vi "testing_cam_ai_ao.vi"() -> ()   [LabVIEW 2015]
uses:
  <vilib>/Platform/storage/lvStorage.llb/_openFunction.ctl
  <vilib>/addons/h5labview2/file/H5Fmode.ctl
  <vilib>/DAQmx/write.llb/DAQmx Write (Analog Wfm 1Chan NSamp).vi
  <vilib>/DAQmx/write.llb/DAQmx Write (Digital Bool 1Line 1Point).vi
  <vilib>/DAQmx/read.llb/DAQmx Read (Analog 1D Wfm NChan NSamp).vi
  <vilib>/DAQmx/create/channels.llb/DAQmx Create Channel (AI-Voltage-Basic).vi
  <vilib>/DAQmx/configure/timing.llb/DAQmx Timing (Sample Clock).vi
  <vilib>/DAQmx/create/channels.llb/DAQmx Create Channel (DO-Digital Output).vi
  <vilib>/DAQmx/create/channels.llb/DAQmx Create Channel (AO-Voltage-Basic).vi
  <vilib>/Platform/storage/lvStorage.llb/_openStorageWithRootAutoDetect.vi
  <vilib>/Platform/storage/lvStorage.llb/xStorage/xStorageSupp/ErrorOut.vi
  <vilib>/Platform/storage/lvStorage.llb/_queryPropPoly.vi
  <vilib>/Platform/storage/lvStorage.llb/_queryPropString.vi
  <vilib>/Platform/storage/lvStorage.llb/_queryGenericObjects.vi
  <vilib>/Platform/storage/lvStorage.llb/_loadAllDdt.vi
  <vilib>/DAQmx/miscellaneous.llb/DAQmx Fill In Error Info.vi
  <vilib>/addons/h5labview2/base/lib_path.vi
  <vilib>/addons/h5labview2/base/H5Equery.vi
  <vilib>/addons/h5labview2/base/hid_t.ctl
  <vilib>/Platform/storage/lvStorage.llb/xStorage/Open Data Storage/Open Data Storage.xnode
  <vilib>/Platform/storage/lvStorage.llb/xStorage/Read Data/Read Data.xnode
  <vilib>/addons/h5labview2/attrib/H5Awrite.llb/H5Awrite.xnode
  <vilib>/addons/h5labview2/dataset/H5Dwrite.llb/H5Dwrite.xnode
  <resource>/objmgr/daqmx.rc
  <vilib>/addons/h5labview2/file/H5F.lvlib
  <vilib>/addons/h5labview2/group/H5G.lvlib
  <vilib>/addons/h5labview2/dataset/H5D.lvlib
  <vilib>/addons/h5labview2/space/H5S.lvlib
panel:
  out "replaced?":bool
  out "error out 4":errorcluster
  out "error out 3":errorcluster
  out "Timeseries Base Filename 2":string
  out "Acquiring Frames":bool
  out "DataPlugin name out":string
  in  "Path":path=path "E:/code/labview-phys-io/001_pure_sines_151013_10Hz.mat"
  out "Actual Sample Rate 2":dbl=1000.0 format="%0.2f"
  out "Stop DAC":bool
  out "n loop":dbl
  out "Measurement":waveform(dbl)[](graph)
  out "error out 2":errorcluster
  out "error out":errorcluster
  in  "Frames":i32=100
  out "Timeseries save path":path
  out "Timeseries Base Filename":string
  out "Image":u16[][](graph)
  in  "stop":bool
  out "Frames Recorded":i32
  in  "Start Button":bool
  out "No Cam Probs":bool
  out "DCAM Ver.":string
  out "Library Ver.":string
  out "Model":string
  out "Camera ID":string
  out "Firmware":string
  out "Actual Sample Rate":dbl=1000.0 format="%0.2f"
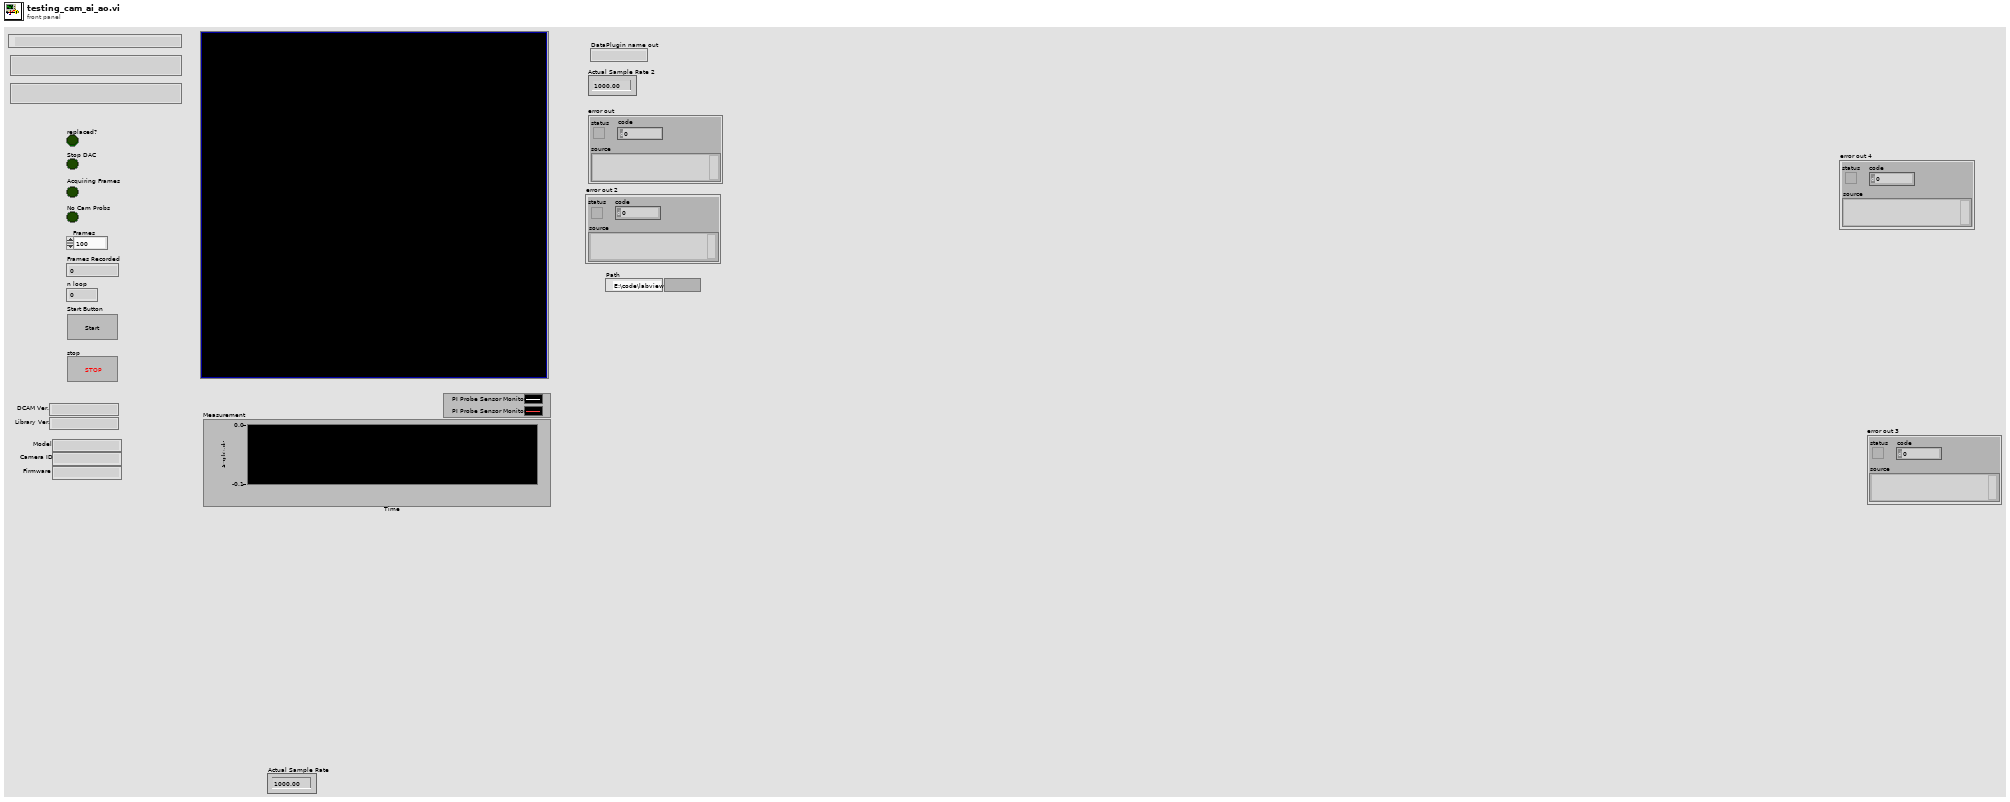
[diagram p1: front panel]
types:
  T1 = cluster{"Capture Library":string, "DCAM-API":string}
  T2 = cluster{"Model":string, "Camera ID":string, "Firmware":string}
  T3 = cluster{"height":u32, "width":u32, "datatype":u32}
  T4 = typedef "H5F.lvlib/H5Fmode.ctl" = enum16{"read-only", "read-write", "overwrite", "create new", "open or create"}
  T5 = typedef "hid_t.ctl" = i32
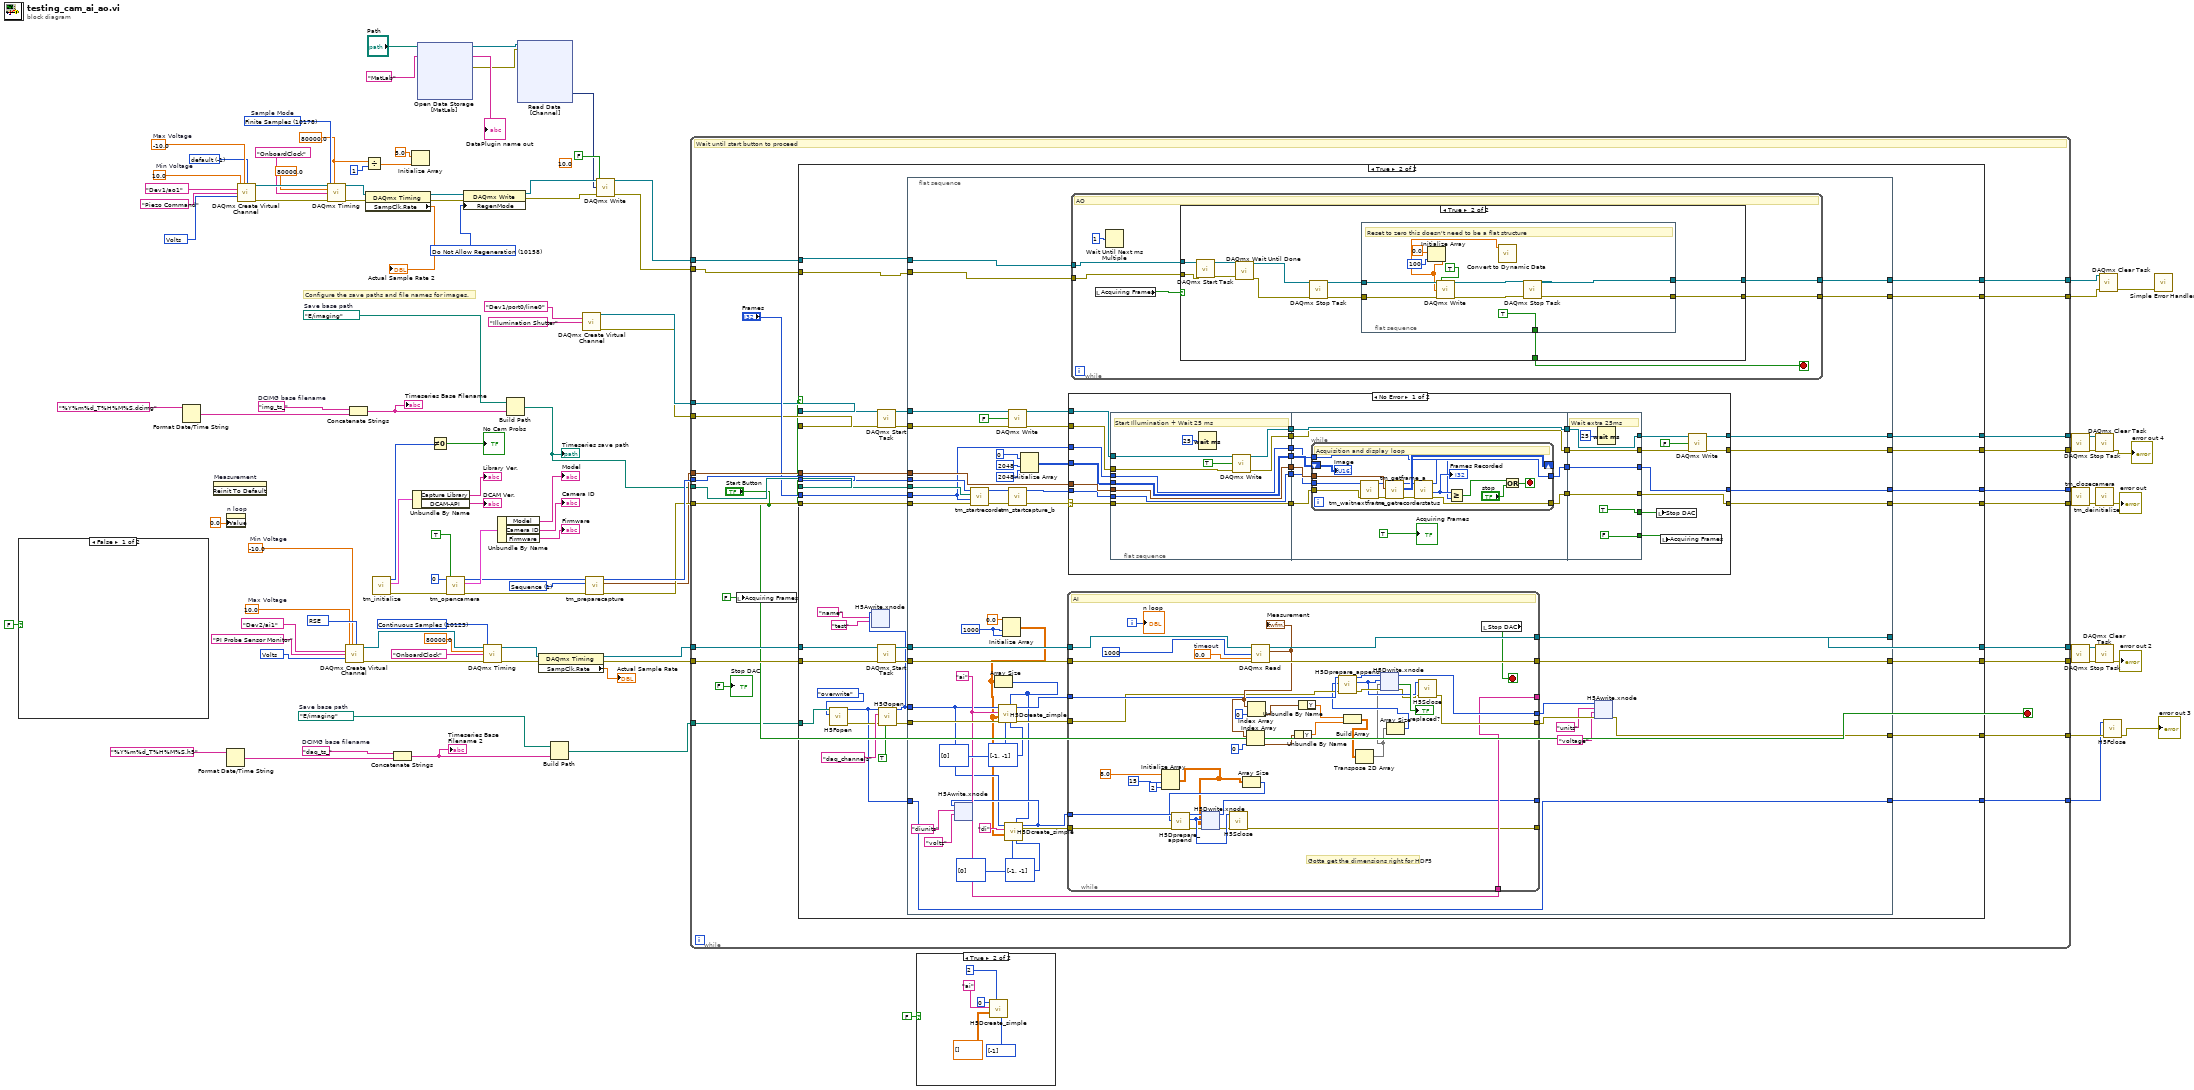
[diagram p0: block diagram]
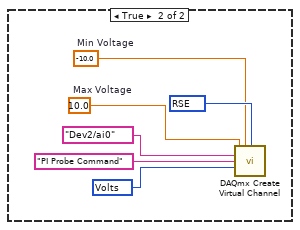
[diagram p3: hidden frame]
diagram:
  w9 = "daq_ts_"  # DCIMG base filename
  w12 = path "E:/imaging"  # Save base path
  w24 = 10158 items=["Allow Regeneration"=10097, "Do Not Allow Regeneration"=10158] ("RegenMode")
  w31 = 80000.0
  (unwired) 10.0
  w38 = 10178 items=["Finite Samples"=10178, "Continuous Samples"=10123, "Hardware Timed Single Point"=12522]  # Sample Mode
  w39 = -1 items=["default"=-1, "RSE"=10083, "NRSE"=10078, "Differential"=10106, "Pseudodifferential"=12529] ("input terminal configuration")
  w40 = 10348 items=["Volts"=10348, "From Custom Scale"=10065] ("units")
  w44 = 10.0  # Min Voltage
  w43 = -10.0  # Max Voltage
  w59 = 1 items=["Snap", "Sequence"] ("Capture mode")
  w67 = 10123 items=["Finite Samples"=10178, "Continuous Samples"=10123] ("sample mode")
  w77 = 10348 items=["Volts"=10348, "From Custom Scale"=10065] ("units")
  w76 = 10083 items=["default"=-1, "RSE"=10083, "NRSE"=10078, "Differential"=10106, "Pseudodifferential"=12529] ("input terminal configuration")
  w74 = -10.0  # Min Voltage
  w75 = 10.0  # Max Voltage
  w91 = "img_ts_"  # DCIMG base filename
  w94 = path "E:/imaging"  # Save base path
  # "Configure the save paths and file names for images."
  n1 = case shown="False" FALSE {
    frame False {
    }
    frame True {
      w109 = 10348 items=["Volts"=10348, "From Custom Scale"=10065] ("units")
      w108 = 10083 items=["default"=-1, "RSE"=10083, "NRSE"=10078, "Differential"=10106, "Pseudodifferential"=12529] ("input terminal configuration")
      w106 = -10.0  # Min Voltage
      w107 = 10.0  # Max Voltage
      n2 = call-poly <vilib>:"DAQmx Create Virtual Channel.vi"("maximum value"=w107, "minimum value"=w106, "input terminal configuration"=w108, "physical channels"=tag "Dev2/ai0" ("DAQmx Physical Channel"), "name to assign"="PI Probe Command", "units"=w109) -> ()  [unwired: 8 in, 2 out]
    }
  }
  n3 = Format Date/Time String(time format string (%c)="%Y%m%d_T%H%M%S.dcimg" ("name or relative path")) -> (date/time string=w92:string)  [unwired: 2 in]
  n4 = invoke on="Measurement" class="WFChart (strict)" method="Reinit To Default"() -> ()  [unwired: 3 in, 3 out]
  n5 = property on="n loop" class="DigNum (strict)"("Value"=0.0 ("n loop")) -> ()  [unwired: 2 in, 2 out]
  n6 = Format Date/Time String(time format string (%c)="%Y%m%d_T%H%M%S.h5" ("name or relative path")) -> (date/time string=w10:string)  [unwired: 2 in]
  n7 = call-poly <vilib>:"DAQmx Create Virtual Channel.vi"("maximum value"=w44, "minimum value"=w43, "output terminal configuration"=w39, "physical channels"=tag "Dev1/ao1" ("DAQmx Physical Channel"), "name to assign"="Piezo Command", "units"=w40) -> ("task out"=w46:refnum<k21>, "error out"=w47:errorcluster)  [unwired: 8 in]
  n8 = call-poly <vilib>:"DAQmx Timing.vi"("task/channels in"=w46, "sample mode"=w38, "samples per channel"=w31, "rate"=80000.0, "source"=tag "OnboardClock" ("Sample Clock Source"), "error in"=w47) -> ("task out"=w36:refnum<k21>, "error out"=w35:errorcluster)  [unwired: 8 in]
  n9 = call-poly <vilib>:"DAQmx Create Virtual Channel.vi"("maximum value"=w75, "minimum value"=w74, "input terminal configuration"=w76, "physical channels"=tag "Dev2/ai1" ("DAQmx Physical Channel"), "name to assign"="PI Probe Sensor Monitor", "units"=w77) -> ("task out"=w69:refnum<k21>, "error out"=w68:errorcluster)  [unwired: 8 in]
  n10 = Concatenate Strings(w91, w92) -> (w90:string)
  "Timeseries Base Filename" <- w90
  n11 = Divide(x=w31, y=1) -> (x/y=w30:dbl)
  n12 = property class="DAQmx Timing"(reference=w36, error in=w35) -> (reference out=w28:refnum<k21>, error out=w27:errorcluster, "SampClk.Rate"=→"Actual Sample Rate 2":dbl)
  n13 = call <userlib>:"tm_initialize.vi"() -> ("error out"=w100:errorcluster, "Version Info"=w104:T1, "Number Of Cameras"=w105:u32)  [unwired: 8 in, 1 out]
  n14 = Concatenate Strings(w9, w10) -> (w8:string)
  "Timeseries Base Filename 2" <- w8
  n15 = Initialize Array(5.0 ("element"), w30) -> ()  [unwired: 1 out]
  n16 = Unbundle By Name(w104) -> ("Capture Library"=→"Library Ver.":string, "DCAM-API"=→"DCAM Ver.":string)
  n17 = xnode "Open Data Storage\n[MatLab]"("file path"="Path", "DataPlugin name"="MatLab") -> ("storage refnum (file)"=w22:refnum<k20>, "DataPlugin name out"=→"DataPlugin name out":string, "error out"=w19:errorcluster)  [unwired: 3 in]
  n18 = Not Equal To 0?(x=w105) -> (x != 0?=→"No Cam Probs":bool)
  n19 = call <userlib>:"tm_opencamera.vi"("Force Open"=TRUE, "error in (no error)"=w100, "Camera Index"=0) -> ("error out"=w57:errorcluster, "Camera Details"=w60:T2, "Handle out"=w58:u32)  [unwired: 6 in]
  n20 = property class="DAQmx Write"(reference=w28, error in=w27, "RegenMode"=w24) -> (reference out=w26:refnum<k21>, error out=w25:errorcluster)
  n21 = call-poly <vilib>:"DAQmx Timing.vi"("task/channels in"=w69, "sample mode"=w67, "rate"=80000.0, "source"=tag "OnboardClock" ("Sample Clock Source"), "error in"=w68) -> ("task out"=w73:refnum<k21>, "error out"=w72:errorcluster)  [unwired: 9 in]
  n22 = Unbundle By Name(w60) -> ("Model"=→"Model":string, "Camera ID"=→"Camera ID":string, "Firmware"=→"Firmware":string)
  n23 = Build Path(base path=w94, name or relative path=w90) -> (appended path=w89:path)
  "Timeseries save path" <- w89
  n24 = xnode "Read Data\n[Channel]"("storage refnum (file)"=w22, "error in"=w19) -> ("Signal"=w20:dynamicdata)  [unwired: 2 in, 3 out]
  n25 = property class="DAQmx Timing"(reference=w73, error in=w72) -> (reference out=w96:refnum<k21>, error out=w95:errorcluster, "SampClk.Rate"=→"Actual Sample Rate":dbl)
  n26 = Build Path(base path=w12, name or relative path=w8) -> (appended path=w7:path)
  n27 = call-poly <vilib>:"DAQmx Create Virtual Channel.vi"("lines"=tag "Dev1/port0/line0" ("DAQmx Physical Channel"), "name to assign"="Illumination Shutter") -> ("task out"=w53:refnum<k21>, "error out"=w52:errorcluster)  [unwired: 12 in]
  n28 = call <userlib>:"tm_preparecapture.vi"("error in (no error)"=w57, "Capture mode"=w59, "Handle in"=w58) -> ("error out"=w98:errorcluster, "Buffer Info"=w97:T3, "Handle out"=w99:u32)  [unwired: 5 in, 1 out]
  n29 = call-poly <vilib>:"DAQmx Write.vi"("task/channels in"=w26, "auto start"=FALSE, "data"=w20, "error in"=w25) -> ("task out"=w17:refnum<k21>, "error out"=w16:errorcluster)  [unwired: 9 in, 1 out]
  n30 = while {
    tunnel: w99 -> [w135]
    tunnel: w98 -> [w133]
    tunnel: w97 -> [w134]
    tunnel: w96 -> [w129]
    tunnel: w95 -> [w128]
    tunnel: w89 -> [w136]
    tunnel: [w131] -> w86
    tunnel: [w130] -> w85
    tunnel: [w127] -> w81
    tunnel: [w126] -> w80
    tunnel: w53 -> [w124]
    tunnel: w52 -> [w123]
    tunnel: [w122] -> w49
    tunnel: [w121] -> w48
    tunnel: w17 -> [w118]
    tunnel: w16 -> [w119]
    tunnel: [w116] -> w14
    tunnel: [w115] -> w13
    tunnel: w7 -> [w114]
    tunnel: [w113] -> w6
    tunnel: [w112] -> w1
    stop <- "Start Button" stop-if-true
    # "Wait until start button to proceed"
    n31 = local write "Acquiring Frames"(FALSE ("Acquiring Frames")) -> ()
    n32 = case shown="True" "Start Button" {
      tunnel: w136 -> [_ w179]
      tunnel: w135 -> [w142 w178]
      tunnel: w134 -> [_ w177]
      tunnel: w133 -> [w141 w176]
      tunnel: "Frames" -> [_ w175]
      tunnel: [w142 w174] -> w131
      tunnel: [w141 w173] -> w130
      tunnel: w129 -> [w144 w172]
      tunnel: w128 -> [w143 w171]
      tunnel: [w144 w168] -> w127
      tunnel: [w143 w167] -> w126
      tunnel: w124 -> [w140 w166]
      tunnel: w123 -> [w139 w165]
      tunnel: [w140 w162] -> w122
      tunnel: [w139 w161] -> w121
      tunnel: w119 -> [w138 w159]
      tunnel: w118 -> [w137 w160]
      tunnel: [w137 w158] -> w116
      tunnel: [w138 w157] -> w115
      tunnel: w114 -> [_ w156]
      tunnel: [_ w154] -> w113
      tunnel: [_ w149] -> w112
      frame False {
      }
      frame True {
        n33 = call <vilib>:"H5Fopen.vi"("mode (read-only)"=H5Fmode."overwrite" ("mode"), "path"=w156) -> ("error out"=w151:errorcluster, "ref out"=w148:T5)  [unwired: 8 in]
        n34 = call <vilib>:"DAQmx Start Task.vi"("task/channels in"=w166, "error in"=w165) -> ("task out"=w163:refnum<k21>, "error out"=w164:errorcluster)  [unwired: 12 in]
        n35 = call <vilib>:"DAQmx Start Task.vi"("task/channels in"=w172, "error in"=w171) -> ("task out"=w170:refnum<k21>, "error out"=w169:errorcluster)  [unwired: 12 in]
        n36 = call <vilib>:"H5Gopen.vi"("create? (F)"=TRUE, "error in (no error)"=w151, "name"="daq_channels", "ref in"=w148) -> ("error out"=w150:errorcluster, "group out"=w147:T5)  [unwired: 6 in]
        n37 = xnode "H5Awrite.xnode"("data"="test" ("name"), "attrib name"="name" ("name"), "ref in"=w147) -> ()  [unwired: 4 in, 3 out]
        n38 = flat-sequence {
          tunnel: w179 -> [w251]
          tunnel: w178 -> [w250]
          tunnel: w177 -> [w249]
          tunnel: w176 -> [w248]
          tunnel: w175 -> [w247]
          tunnel: w170 -> [w236]
          tunnel: w169 -> [w235]
          tunnel: w163 -> [w231]
          tunnel: w164 -> [w230]
          tunnel: [w246] -> w174
          tunnel: [w245] -> w173
          tunnel: [w234] -> w168
          tunnel: [w233] -> w167
          tunnel: [w227] -> w162
          tunnel: [w226] -> w161
          tunnel: w159 -> [w225]
          tunnel: w160 -> [w224]
          tunnel: [w223] -> w158
          tunnel: [w222] -> w157
          tunnel: w150 -> [w213]
          tunnel: [w219] -> w154
          tunnel: w148 -> [w216]
          tunnel: [w216] -> w149
          tunnel: w147 -> [w201]
          frame #0 {
            w200 = 1000 ("dimension size")
            w211 = "ai"
            n39 = call <userlib>:"tm_startrecorder.vi"("error in (no error)"=w248, "frames"=w247, "File"=w251, "Handle in"=w250) -> ("error out"=w239:errorcluster, "Handle out"=w238:u32)  [unwired: 6 in]
            n40 = Initialize Array(0.0 ("element"), w200, w200) -> (w199:dbl[][])
            n41 = Array Size(array=w199) -> (size(s)=w198:i32[])
            n42 = call <vilib>:"H5Dcreate_simple.vi"("max size"=i32[] [-1, -1], "chunk size"=w198, "initial size"=i32[] [0], "error in (no error)"=w213, "type in"=w199, "name"=w211, "ref in"=w201) -> ("error out"=w202:errorcluster, "dset out"=w212:T5)  [unwired: 3 in]
            n43 = call <vilib>:"H5Dcreate_simple.vi"("max size"=i32[] [-1, -1], "chunk size"=w198, "initial size"=i32[] [0], "type in"=w199, "name"="di", "ref in"=w201) -> ("error out"=w206:errorcluster, "dset out"=w203:T5)  [unwired: 4 in]
            n44 = xnode "H5Awrite.xnode"("data"="voltz" ("name"), "attrib name"="diunits" ("name"), "ref in"=w203) -> ()  [unwired: 4 in, 3 out]
            n45 = call-poly <vilib>:"DAQmx Write.vi"("task/channels in"=w231, "data"=FALSE, "error in"=w230) -> ("task out"=w229:refnum<k21>, "error out"=w228:errorcluster)  [unwired: 10 in, 1 out]
            n46 = call <userlib>:"tm_startcapture_b.vi"("error in (no error)"=w239, "Handle in"=w238) -> ("error out"=w237:errorcluster, "Handle out"=w244:u32)  [unwired: 8 in]
            n47 = Initialize Array(u16 0 ("element"), 2048 ("dimension size"), 2048 ("dimension size")) -> (w240:u16[][])
            n48 = while {
              tunnel: w235 -> [w359]
              tunnel: w236 -> [w358]
              tunnel: [w357] -> w234
              tunnel: [w356] -> w233
              tunnel: [w337] -> _
              tunnel: [w342] -> w220
              tunnel: [w340] -> w221
              tunnel: w212 -> [w339]
              tunnel: w202 -> [w338]
              tunnel: w211 -> [w337]
              tunnel: w206 -> [w332]
              tunnel: w203 -> [w331]
              tunnel: [w329] -> _
              tunnel: [w328] -> _
              i -> [w352]
              stop <- w353 stop-if-true
              w355 = 0.0  # timeout
              # "Gotta get the dimensions right for HDF5"
              # "AI"
              n49 = Initialize Array(8.0 ("element"), 15 ("dimension size"), 2 ("dimension size")) -> (w319:dbl[][])
              n50 = Array Size(array=w319) -> (size(s)=w322:i32[])
              n51 = call <vilib>:"H5Dprepare_append.vi"("error in (no error)"=w332, "append dims"=w322, "dset in"=w331) -> ("error out"=w333:errorcluster, "space out"=w335:T5, "dset out"=w336:T5)  [unwired: 6 in]
              n52 = xnode "H5Dwrite.xnode"("error in (no error)"=w333, "data"=w319, "file space"=w335, "ref in"=w336) -> ("error out"=w334:errorcluster, "ref out"=w329:T5)  [unwired: 3 in, 1 out]
              n53 = call <vilib>:"H5Sclose.vi"("error in (no error)"=w334, "space in"=w335) -> ("error out"=w328:errorcluster)  [unwired: 9 in]
              n54 = call-poly <vilib>:"DAQmx Read.vi"("task/channels in"=w358, "number of samples per channel"=1000 ("Samples to Read"), "timeout"=w355, "error in"=w359) -> ("task out"=w357:refnum<k21>, "data"=w348:waveform(dbl)[], "error out"=w356:errorcluster)  [unwired: 9 in]
              "Measurement" <- w348
              n55 = Index Array(array=w348, index=0) -> (element=w347:waveform(dbl))
              n56 = Index Array(array=w348, index=0) -> (element=w350:waveform(dbl))
              n57 = Unbundle By Name(w347) -> ("Y"=w326:dbl[])
              n58 = Unbundle By Name(w350) -> ("Y"=w327:dbl[])
              n59 = Build Array(w327, w326) -> (w324:dbl[][])
              n60 = Transpose 2D Array(2D array=w324) -> (transposed array=w323:dbl[][])
              n61 = Array Size(array=w323) -> (size(s)=w325:i32[])
              n62 = call <vilib>:"H5Dprepare_append.vi"("error in (no error)"=w338, "append dims"=w325, "dset in"=w339) -> ("error out"=w344:errorcluster, "space out"=w343:T5, "dset out"=w345:T5)  [unwired: 6 in]
              n63 = xnode "H5Dwrite.xnode"("error in (no error)"=w344, "data"=w323, "file space"=w343, "ref in"=w345) -> ("error out"=w341:errorcluster, "replaced?"=→"replaced?":bool, "ref out"=w342:T5)  [unwired: 3 in]
              n64 = call <vilib>:"H5Sclose.vi"("error in (no error)"=w341, "space in"=w343) -> ("error out"=w340:errorcluster)  [unwired: 9 in]
              n65 = local read "Stop DAC"() -> (w353:bool)
              "n loop" <- w352
            }
            n66 = case shown="No Error" w237 {
              selector: w237 -> [w416 w470]
              tunnel: w249 -> [w422 _]
              tunnel: w244 -> [w421 w469]
              tunnel: w240 -> [w420 _]
              tunnel: [w419 w469] -> w246
              tunnel: [w418 w470] -> w245
              tunnel: w247 -> [w417 _]
              tunnel: w229 -> [w407 w467]
              tunnel: w228 -> [w406 w468]
              tunnel: [w398 w467] -> w227
              tunnel: [w397 w468] -> w226
              frame No Error {
                n67 = flat-sequence {
                  tunnel: w416 -> [w429]
                  tunnel: w417 -> [w430]
                  tunnel: w420 -> [w431]
                  tunnel: w421 -> [w432]
                  tunnel: w422 -> [w433]
                  tunnel: [w433] -> w412
                  tunnel: [w432] -> w411
                  tunnel: [w431] -> w410
                  tunnel: [w430] -> w409
                  tunnel: [w429] -> w408
                  tunnel: w407 -> [w426]
                  tunnel: w406 -> [w425]
                  tunnel: [w424] -> w404
                  tunnel: [w423] -> w399
                  tunnel: [w440] -> w414
                  tunnel: [w439] -> w413
                  tunnel: w412 -> [w443]
                  tunnel: w411 -> [w442]
                  tunnel: w410 -> [w441]
                  tunnel: w409 -> [w438]
                  tunnel: w408 -> [w437]
                  tunnel: w404 -> [w436]
                  tunnel: [w436] -> w403
                  tunnel: [w435] -> w400
                  tunnel: w399 -> [w435]
                  tunnel: [TRUE] -> w415
                  tunnel: [w465] -> w418
                  tunnel: [w466] -> w419
                  tunnel: w414 -> [w466]
                  tunnel: w413 -> [w465]
                  tunnel: w403 -> [w462]
                  tunnel: [w462] -> w402
                  tunnel: [w461] -> w401
                  tunnel: w400 -> [w461]
                  tunnel: [FALSE] -> w396
                  frame #0 {
                    # "Start Illumination + Wait 25 ms"
                    n68 = Wait (ms)(milliseconds to wait=u32 25) -> ()  [unwired: 1 out]
                    n69 = call-poly <vilib>:"DAQmx Write.vi"("task/channels in"=w426, "data"=TRUE, "error in"=w425) -> ("task out"=w424:refnum<k21>, "error out"=w423:errorcluster)  [unwired: 10 in, 1 out]
                  }
                  frame #1 {
                    n70 = while {
                      tunnel: w443 -> [w459]
                      tunnel: w442 -> [w458]
                      tunnel: w437 -> [w455]
                      shift-right: [w453] -> _
                      shift-left: w441 -> [w454]
                      tunnel: [w450] -> w440
                      tunnel: [w449] -> w439
                      tunnel: w438 -> [w444]
                      stop <- w447 stop-if-true
                      # "Acquisition and display loop"
                      n71 = call <userlib>:"tm_waitnextframe.vi"("error in (no error)"=w455, "Handle in"=w458) -> ("error out"=w456:errorcluster, "Handle out"=w457:u32)  [unwired: 6 in, 2 out]
                      n72 = call <userlib>:"tm_getframe_a.vi"("error in (no error)"=w456, "Buffer Info"=w459, "Handle in"=w457) -> ("error out"=w452:errorcluster, "Data 16"=w453:u16[][], "Handle out"=w451:u32)  [unwired: 4 in, 2 out]
                      n73 = call <userlib>:"tm_getrecorderstatus.vi"("error in (no error)"=w452, "Handle"=w451) -> ("error out"=w449:errorcluster, "Count"=w445:i32, "Handle"=w450:u32)  [unwired: 6 in, 1 out]
                      "Frames Recorded" <- w445
                      n74 = Greater Or Equal?(x=w445, y=w444) -> (x >= y?=w446:bool)
                      n75 = Or(x=w446, y="stop") -> (x .or. y?=w447:bool)
                      "Image" <- w454
                    }
                    "Acquiring Frames" <- TRUE
                  }
                  frame #2 {
                    # "Wait extra 25ms"
                    n76 = Wait (ms)(milliseconds to wait=u32 25) -> ()  [unwired: 1 out]
                  }
                }
                n77 = local write "Stop DAC"(w415) -> ()
                n78 = local write "Acquiring Frames"(w396) -> ()
                n79 = call-poly <vilib>:"DAQmx Write.vi"("task/channels in"=w402, "data"=FALSE, "error in"=w401) -> ("task out"=w398:refnum<k21>, "error out"=w397:errorcluster)  [unwired: 10 in, 1 out]
              }
              frame Error {
              }
            }
            n80 = while {
              tunnel: w225 -> [w292]
              tunnel: w224 -> [w293]
              tunnel: [w289] -> w223
              tunnel: [w288] -> w222
              stop <- w291 stop-if-true
              # "AO"
              n81 = local read "Acquiring Frames"() -> (w290:bool)
              n82 = Wait Until Next ms Multiple(millisecond multiple=u32 1) -> ()  [unwired: 1 out]
              n83 = case shown="True" w290 {
                tunnel: w293 -> [w296 w307]
                tunnel: w292 -> [w295 w306]
                tunnel: [_ w305] -> w291
                tunnel: [w296 w298] -> w289
                tunnel: [w295 w297] -> w288
                frame False {
                }
                frame True {
                  n84 = call <vilib>:"DAQmx Start Task.vi"("task/channels in"=w307, "error in"=w306) -> ("task out"=w304:refnum<k21>, "error out"=w303:errorcluster)  [unwired: 12 in]
                  n85 = call <vilib>:"DAQmx Wait Until Done.vi"("task/channels in"=w304, "error in"=w303) -> ("task out"=w301:refnum<k21>, "error out"=w302:errorcluster)  [unwired: 12 in]
                  n86 = call <vilib>:"DAQmx Stop Task.vi"("task/channels in"=w301, "error in"=w302) -> ("task out"=w299:refnum<k21>, "error out"=w300:errorcluster)  [unwired: 12 in]
                  n87 = flat-sequence {
                    tunnel: w299 -> [w317]
                    tunnel: w300 -> [w312]
                    tunnel: [TRUE] -> w305
                    tunnel: [w311] -> w298
                    tunnel: [w310] -> w297
                    frame #0 {
                      # "Reset to zero this doesn't need to be a flat structure"
                      n88 = Initialize Array(0.0 ("element"), 100 ("dimension size")) -> (w313:dbl[])
                      n89 = call-poly <vilib>:"DAQmx Write.vi"("task/channels in"=w317, "auto start"=TRUE, "data"=w313, "error in"=w312) -> ("task out"=w309:refnum<k21>, "error out"=w308:errorcluster)  [unwired: 9 in, 1 out]
                      n90 = call "Convert to Dynamic Data"("Array"=w313) -> ()  [unwired: 3 in, 1 out]
                      n91 = call <vilib>:"DAQmx Stop Task.vi"("task/channels in"=w309, "error in"=w308) -> ("task out"=w311:refnum<k21>, "error out"=w310:errorcluster)  [unwired: 12 in]
                    }
                  }
                }
              }
            }
            n92 = xnode "H5Awrite.xnode"("error in (no error)"=w221, "data"="voltage" ("name"), "attrib name"="units" ("name"), "ref in"=w220) -> ("error out"=w219:errorcluster)  [unwired: 3 in, 2 out]
          }
        }
      }
    }
    "Stop DAC" <- FALSE
  }
  n93 = case shown="True" FALSE {
    frame False {
    }
    frame True {
      n94 = call <vilib>:"H5Dcreate_simple.vi"("max size"=i32[] [-1], "ndims"=2, "type in"=dbl[][] [], "name"="ai", "ref in"=T5 0) -> ()  [unwired: 5 in, 2 out]
    }
  }
  n95 = call <vilib>:"DAQmx Stop Task.vi"("task/channels in"=w49, "error in"=w48) -> ("task out"=w51:refnum<k21>, "error out"=w50:errorcluster)  [unwired: 12 in]
  n96 = call <userlib>:"tm_closecamera.vi"("error in (no error)"=w85, "Handle in"=w86) -> ("error out"=w87:errorcluster)  [unwired: 9 in]
  n97 = call <vilib>:"DAQmx Stop Task.vi"("task/channels in"=w81, "error in"=w80) -> ("task out"=w84:refnum<k21>, "error out"=w83:errorcluster)  [unwired: 12 in]
  n98 = call <vilib>:"DAQmx Clear Task.vi"("task in"=w51, "error in"=w50) -> ("error out"=→"error out 4":errorcluster)  [unwired: 13 in]
  n99 = call <userlib>:"tm_deinitialize.vi"("error in (no error)"=w87) -> ("error out"=→"error out":errorcluster)  [unwired: 10 in]
  n100 = call <vilib>:"DAQmx Clear Task.vi"("task in"=w84, "error in"=w83) -> ("error out"=→"error out 2":errorcluster)  [unwired: 13 in]
  n101 = call <vilib>:"DAQmx Clear Task.vi"("task in"=w14, "error in"=w13) -> ("error out"=w15:errorcluster)  [unwired: 13 in]
  n102 = call <vilib>:"H5Fclose.vi"("error in (no error)"=w6, "ref"=w1) -> ("error out"=→"error out 3":errorcluster)  [unwired: 9 in]
  n103 = call <vilib>:"Simple Error Handler.vi"("error in (no error)"=w15) -> ()  [unwired: 4 in, 5 out]
